vi "For Loop+Indicators Count Up and Down.vi"() -> ()   [LabVIEW 2019]
panel:
  out "Count Up to 30":dbl(knob) scale=0.0..30.0
  out "Count Down from 30":dbl(slide)=30.0 scale=0.0..30.0
  # "Challenge:\nCount Up, Count Down. Create two different indicators on the front panel, one that counts up to 30 at one-second intervals and one that counts down from 30 at the same time."
  # "Try it: Run the program and watch the up and down counters."
  # "You will probably need:\nIndicators, for loops, wait for ms, numeric functions"
  # "Open the block diagram to see a possible solution."
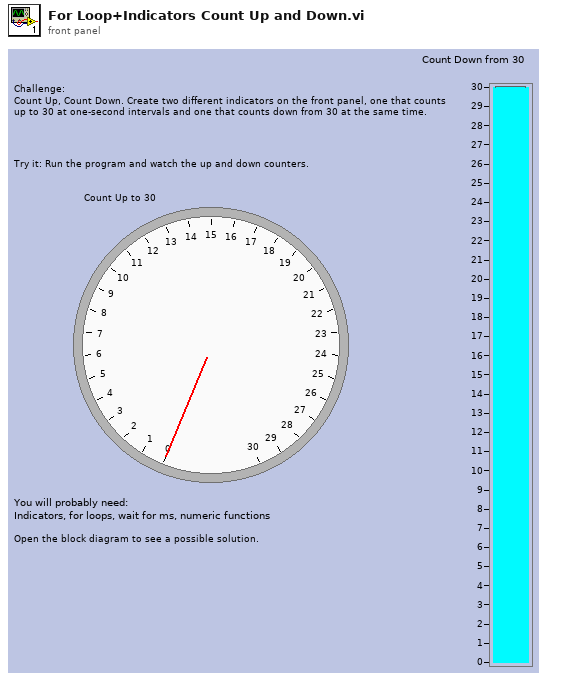
[diagram p1: front panel]
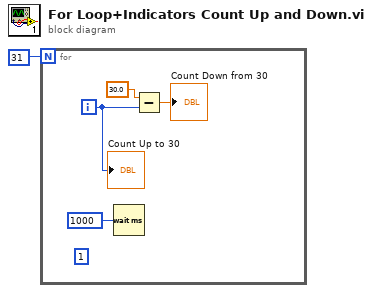
[diagram p0: block diagram]
diagram:
  n1 = for {
    N: 31 -> [_]
    i -> [w2]
    (unwired) 1
    n2 = Wait (ms)(milliseconds to wait=1000) -> ()  [unwired: 1 out]
    n3 = Subtract(x=30.0 ("y"), y=w2) -> (x-y=→"Count Down from 30":dbl)
    "Count Up to 30" <- w2
  }
